vi "Main.vi"(8 "error in (no error)":errorcluster, 11 "Plugin Thread in":refnum<class "Plugin Thread.lvclass">) -> (0 "error out":errorcluster, 3 "Plugin Thread out":refnum<class "Plugin Thread.lvclass">)   [LabVIEW 2019, in "DSF Core.lvlib" / "Plugin Thread.lvclass"]
uses:
  Thread/Plugin/Plugin Thread.lvclass
  Thread/Thread.lvclass
  Transfer Group/Transfer Group.lvclass
  C:/Dev/GitHub/niveristand-data-sharing-framework-custom-device/Core/Classes/Thread/Thread.lvclass
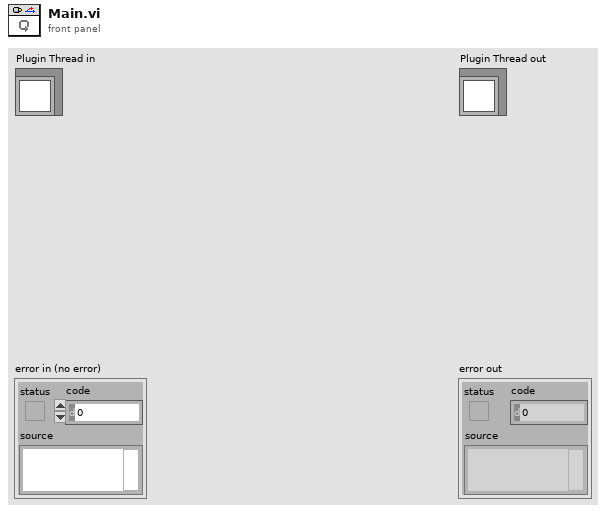
[diagram p1: front panel]
types:
  T1 = typedef "DSF Core.lvlib/Plugin Thread.lvclass/Command Data.ctl" = cluster{"Command":T2, "Parameters":T3}
  T2 = typedef "DSF Core.lvlib/Plugin Thread.lvclass/Commands.ctl" = enum8{"Idle", "Error", "Start", "Rx", "Tx", "Shutdown"}
  T3 = typedef "DSF Core.lvlib/Plugin Interface.lvclass/Command Parameters.ctl" = cluster{"arg1":u64, "arg2":u64}
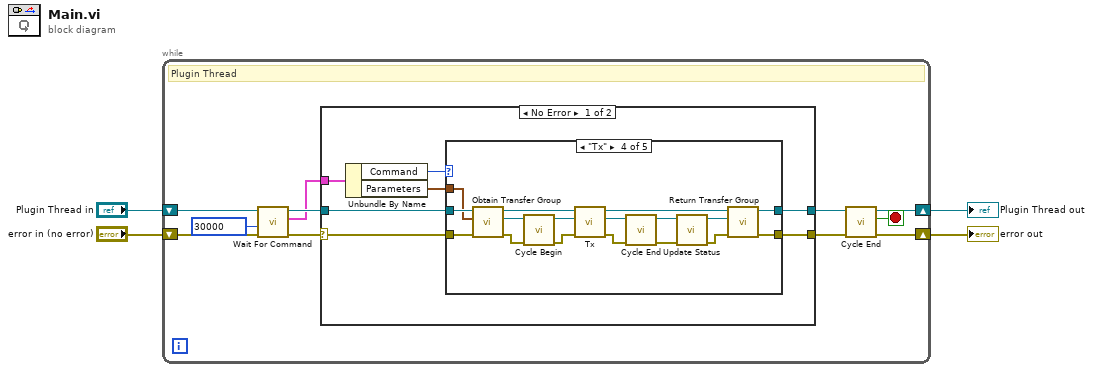
[diagram p0: block diagram]
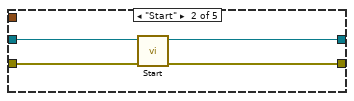
[diagram p3: hidden frame]
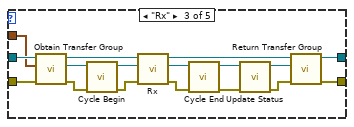
[diagram p4: hidden frame]
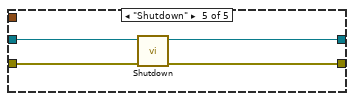
[diagram p5: hidden frame]
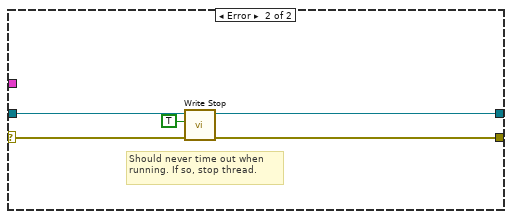
[diagram p6: hidden frame]
diagram:
  n1 = while {
    shift-right: [w6] -> w3
    shift-left: "error in (no error)" -> [w15]
    shift-right: [w7] -> w2
    shift-left: "Plugin Thread in" -> [w14]
    stop <- w5 stop-if-true
    # "Plugin Thread"
    n2 = call "Wait For Command.vi"("error in (no error)"=w15, "timeout in ms (0)"=30000 ("timeout in ms"), "Plugin Thread in"=w14) -> ("error out"=w11:errorcluster, "command"=w10:T1, "Plugin Thread out"=w12:refnum<class "Plugin Thread.lvclass">)  [unwired: 6 in]
    n3 = case shown="No Error" w11 {
      selector: w11 -> [w19 w70]
      tunnel: w12 -> [w20 w71]
      tunnel: [w22 w67] -> w9
      tunnel: w10 -> [w18 _]
      tunnel: [w21 w69] -> w8
      frame No Error {
        n4 = Unbundle By Name(w18) -> ("Command"=w17:T2, "Parameters"=w16:T3)
        n5 = case shown="\"Tx\"" w17 {
          tunnel: w20 -> [w24 w28 w45 w62 w66]
          tunnel: [w24 w26 w42 w59 w64] -> w22
          tunnel: w19 -> [w23 w27 w43 w61 w65]
          tunnel: w16 -> [_ _ w44 w60 _]
          tunnel: [w23 w25 w41 w58 w63] -> w21
          frame "Idle", "Error" {
          }
          frame "Start" {
            n6 = call-dynamic "Start.vi"("error in (no error)"=w27, "Plugin Thread in"=w28) -> ("error out"=w25:errorcluster, "Plugin Thread out"=w26:refnum<class "Plugin Thread.lvclass">)  [unwired: 8 in]
          }
          frame "Rx" {
            n7 = call "Obtain Transfer Group.vi"("error in (no error)"=w43, "command parameters"=w44, "Transceiver Thread in"=w45) -> ("error out"=w37:errorcluster, "Transfer Group"=w38:refnum<class "Transfer Group.lvclass">, "Transceiver Thread out"=w40:refnum<class "Plugin Thread.lvclass">)  [unwired: 6 in]
            n8 = call "Cycle Begin.vi"("error in (no error)"=w37, "Transfer Group in"=w38) -> ("error out"=w35:errorcluster, "Transfer Group out"=w36:refnum<class "Transfer Group.lvclass">)  [unwired: 8 in]
            n9 = call-dynamic "Rx.vi"("error in (no error)"=w35, "Transfer Group in"=w36, "Plugin Thread in"=w40) -> ("error out"=w33:errorcluster, "Transfer Group out"=w34:refnum<class "Transfer Group.lvclass">, "Plugin Thread out"=w39:refnum<class "Plugin Thread.lvclass">)  [unwired: 6 in]
            n10 = call "Cycle End.vi"("error in (no error)"=w33, "Transfer Group in"=w34) -> ("error out"=w32:errorcluster, "Transfer Group out"=w31:refnum<class "Transfer Group.lvclass">)  [unwired: 8 in]
            n11 = call "Update Status.vi"("error in (no error)"=w32, "Transfer Group in"=w31) -> ("error out"=w30:errorcluster, "Transfer Group out"=w29:refnum<class "Transfer Group.lvclass">)  [unwired: 8 in]
            n12 = call "Return Transfer Group.vi"("error in (no error)"=w30, "Transfer Group in"=w29, "Transceiver Thread in"=w39) -> ("error out"=w41:errorcluster, "Transceiver Thread out"=w42:refnum<class "Plugin Thread.lvclass">)  [unwired: 7 in]
          }
          frame "Tx" {
            n13 = call "Obtain Transfer Group.vi"("error in (no error)"=w61, "command parameters"=w60, "Transceiver Thread in"=w62) -> ("error out"=w52:errorcluster, "Transfer Group"=w55:refnum<class "Transfer Group.lvclass">, "Transceiver Thread out"=w57:refnum<class "Plugin Thread.lvclass">)  [unwired: 6 in]
            n14 = call "Cycle Begin.vi"("error in (no error)"=w52, "Transfer Group in"=w55) -> ("error out"=w51:errorcluster, "Transfer Group out"=w50:refnum<class "Transfer Group.lvclass">)  [unwired: 8 in]
            n15 = call-dynamic "Tx.vi"("error in (no error)"=w51, "Transfer Group in"=w50, "Plugin Thread in"=w57) -> ("error out"=w53:errorcluster, "Transfer Group out"=w54:refnum<class "Transfer Group.lvclass">, "Plugin Thread out"=w56:refnum<class "Plugin Thread.lvclass">)  [unwired: 6 in]
            n16 = call "Cycle End.vi"("error in (no error)"=w53, "Transfer Group in"=w54) -> ("error out"=w49:errorcluster, "Transfer Group out"=w48:refnum<class "Transfer Group.lvclass">)  [unwired: 8 in]
            n17 = call "Update Status.vi"("error in (no error)"=w49, "Transfer Group in"=w48) -> ("error out"=w47:errorcluster, "Transfer Group out"=w46:refnum<class "Transfer Group.lvclass">)  [unwired: 8 in]
            n18 = call "Return Transfer Group.vi"("error in (no error)"=w47, "Transfer Group in"=w46, "Transceiver Thread in"=w56) -> ("error out"=w58:errorcluster, "Transceiver Thread out"=w59:refnum<class "Plugin Thread.lvclass">)  [unwired: 7 in]
          }
          frame "Shutdown" {
            n19 = call-dynamic "Shutdown.vi"("error in (no error)"=w65, "Plugin Thread in"=w66) -> ("error out"=w63:errorcluster, "Plugin Thread out"=w64:refnum<class "Plugin Thread.lvclass">)  [unwired: 8 in]
          }
        }
      }
      frame Error {
        # "Should never time out when running. If so, stop thread."
        n20 = call "Write Stop.vi"("error in (no error)"=w70, "stop"=TRUE, "Thread in"=w71) -> ("error out"=w69:errorcluster, "Thread out"=w67:refnum<class "Plugin Thread.lvclass">)  [unwired: 7 in]
      }
    }
    n21 = call "Cycle End.vi"("error in (no error)"=w8, "Plugin Thread in"=w9) -> ("error out"=w6:errorcluster, "stop"=w5:bool, "Plugin Thread out"=w7:refnum<class "Plugin Thread.lvclass">)  [unwired: 7 in]
  }
  "error out" <- w3
  "Plugin Thread out" <- w2
